vi "flatten gains.vi"(8 "derivative time (Td, min)":dbl, 9 "integral time (Ti, min)":dbl, 10 "proportional gain (Kc)":dbl, 11 "ID":string) -> (3 "wrapped data":string)   [LabVIEW 2013, in "PID Loop.lvclass"]
uses:
  PID Loop.lvclass
  String Parameters.ctl
  <vilib>/NI/Configuration Framework/serializable configuration/NISE_CEF_serializable configuration.lvclass
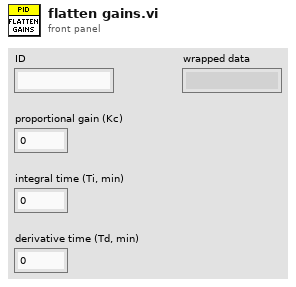
[diagram p1: front panel]
types:
  T1 = typedef "PID Loop.lvclass/String Parameters.ctl" = enum16{"Setpoint", "Process Variable", "Output", "Proportional Gain", "Integral Time", "Derivative Time", "Range High", "Range Low"}
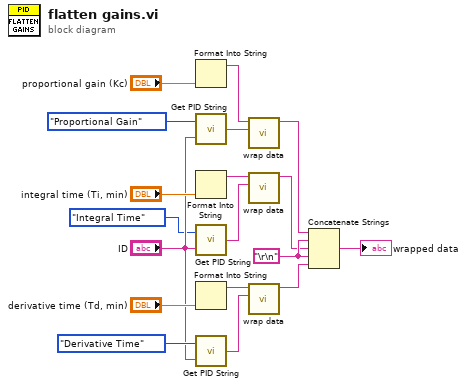
[diagram p0: block diagram]
diagram:
  w17 = "\r\n"
  n1 = Format Into String("proportional gain (Kc)") -> (resulting string=w6:string)  [unwired: 3 in, 1 out]
  n2 = call "Get PID String.vi"("PID Loop ID"="ID", "PID Parameter"=String_Parameters."Proportional Gain") -> ("Parameter String"=w5:string)
  n3 = Format Into String("integral time (Ti, min)") -> (resulting string=w8:string)  [unwired: 3 in, 1 out]
  n4 = call "Get PID String.vi"("PID Loop ID"="ID", "PID Parameter"=String_Parameters."Integral Time") -> ("Parameter String"=w9:string)
  n5 = Format Into String("derivative time (Td, min)") -> (resulting string=w16:string)  [unwired: 3 in, 1 out]
  n6 = call "Get PID String.vi"("PID Loop ID"="ID", "PID Parameter"=String_Parameters."Derivative Time") -> ("Parameter String"=w10:string)
  n7 = call <vilib>:"wrap data.vi"("identifier"=w5, "data to wrap"=w6) -> ("wrapped data"=w3:string)  [unwired: 9 in]
  n8 = call <vilib>:"wrap data.vi"("identifier"=w9, "data to wrap"=w8) -> ("wrapped data"=w2:string)  [unwired: 9 in]
  n9 = call <vilib>:"wrap data.vi"("identifier"=w10, "data to wrap"=w16) -> ("wrapped data"=w18:string)  [unwired: 9 in]
  n10 = Concatenate Strings(w3, w17, w2, w17, w18) -> (→"wrapped data":string)
